vi "Display Message.vi"(6 "Enable Lower Message (T: Enable)":bool=TRUE, 7 "Enable Upper Message (T: Enable)":bool=TRUE, 8 "error in (no error)":errorcluster, 9 "Lower Message (\"Message\")":string="Message", 10 "Upper Message (\"Default\")":string="Default", 11 "VISA resource name":refnum<visa-resource-name>) -> (0 "error out":errorcluster, 3 "VISA resource name out":refnum<visa-resource-name>)   [LabVIEW 2017, in "Keithley 24XX.lvlib"]
doc: "Displays a message on the instrument's display."
uses:
  Keithley 24XX.lvlib
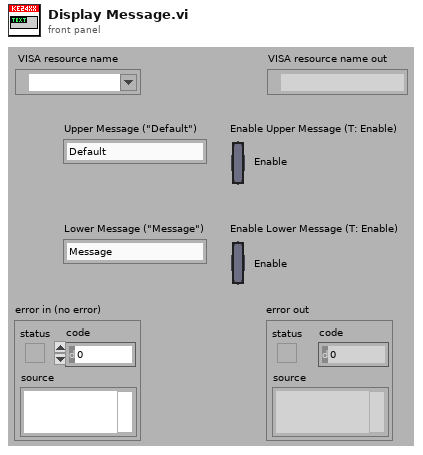
[diagram p1: front panel]
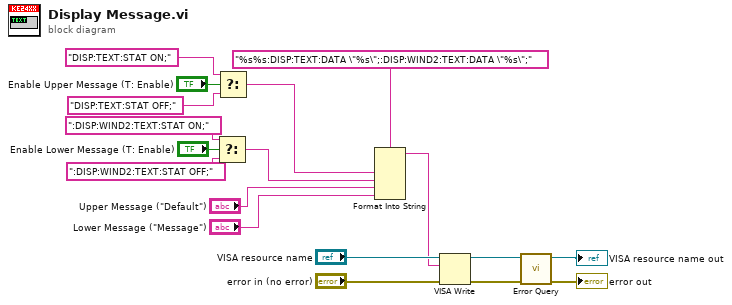
[diagram p0: block diagram]
diagram:
  n1 = Select(t=":DISP:WIND2:TEXT:STAT ON;", s="Enable Lower Message (T: Enable)", f=":DISP:WIND2:TEXT:STAT OFF;") -> (s? t:f=w3:string)
  n2 = Select(t="DISP:TEXT:STAT ON;", s="Enable Upper Message (T: Enable)", f="DISP:TEXT:STAT OFF;") -> (s? t:f=w4:string)
  n3 = Format Into String(format string="%s%s:DISP:TEXT:DATA \"%s\";:DISP:WIND2:TEXT:DATA \"%s\";", w4, w3, "Upper Message (\"Default\")", "Lower Message (\"Message\")") -> (resulting string=w12:string)  [unwired: 2 in, 1 out]
  n4 = VISA Write(VISA resource name="VISA resource name", write buffer=w12, error in (no error)="error in (no error)") -> (VISA resource name out=w16:refnum<visa-resource-name>, error out=w13:errorcluster)  [unwired: 1 out]
  n5 = call "Error Query.vi"("error in (no error)"=w13, "VISA resource name"=w16) -> ("error out"=→"error out":errorcluster, "VISA resource name out"=→"VISA resource name out":refnum<visa-resource-name>)  [unwired: 6 in, 2 out]
